vi "Inverter-data-vi.vi"() -> ()   [LabVIEW 2016]
uses:
  <vilib>/Modbus/subvis/Modbus API/Modbus API.lvclass/Modbus API.ctl
  <vilib>/Modbus/subvis/Transmission Data Unit (ADU)/Transmission Data Unit/Transmission Data Unit.lvclass/Transmission Data Unit.ctl
  <vilib>/Modbus/master/Data Access/Unit ID/Set Unit ID Property.vi
  <vilib>/Modbus/subvis/Transmission Data Unit (ADU)/Transmission Data Unit/Data Access/Unit ID/Write Unit ID.vi
  <vilib>/Modbus/subvis/Modbus API/Read Transmission Data Unit.vi
  <vilib>/Modbus/subvis/Modbus API/Write Transmission Data Unit.vi
  <vilib>/Modbus/master/Modbus Master.lvclass
  C:/Program Files (x86)/National Instruments/LabVIEW 2016/vi.lib/Modbus/subvis/Modbus API/Modbus API.lvclass
  <vilib>/Modbus/master/Create Master Instance (TCP).vi
  <vilib>/Modbus/subvis/Transmission Data Unit (ADU)/Transmission Data Unit/Transmission Data Unit.lvclass
panel:
  in  "INVERTER IP: 192.168.0.151":string
  in  "error in (no error)":errorcluster
  out "error out":errorcluster
  in  "Unit ID":u8
  in  "number of holding registers":u32
  out "BATT-TEMP":dbl
  out "DC-VOLT":dbl
  out "AC-LOAD VOLTAGE":dbl
  out "AC-LOAD-CURRENT":dbl
  out "AC-LOAD-POWER":dbl
  out "INVERTER DATA":cluster{dbl[], dbl[]}[](graph)
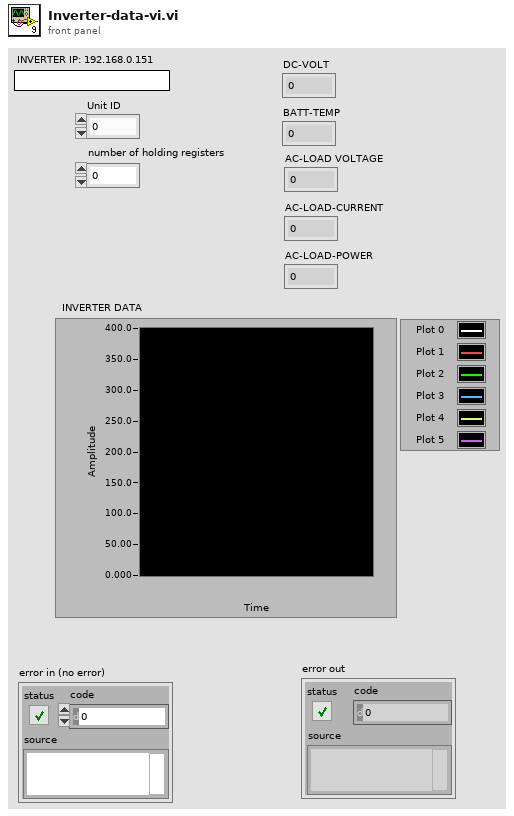
[diagram p1: front panel]
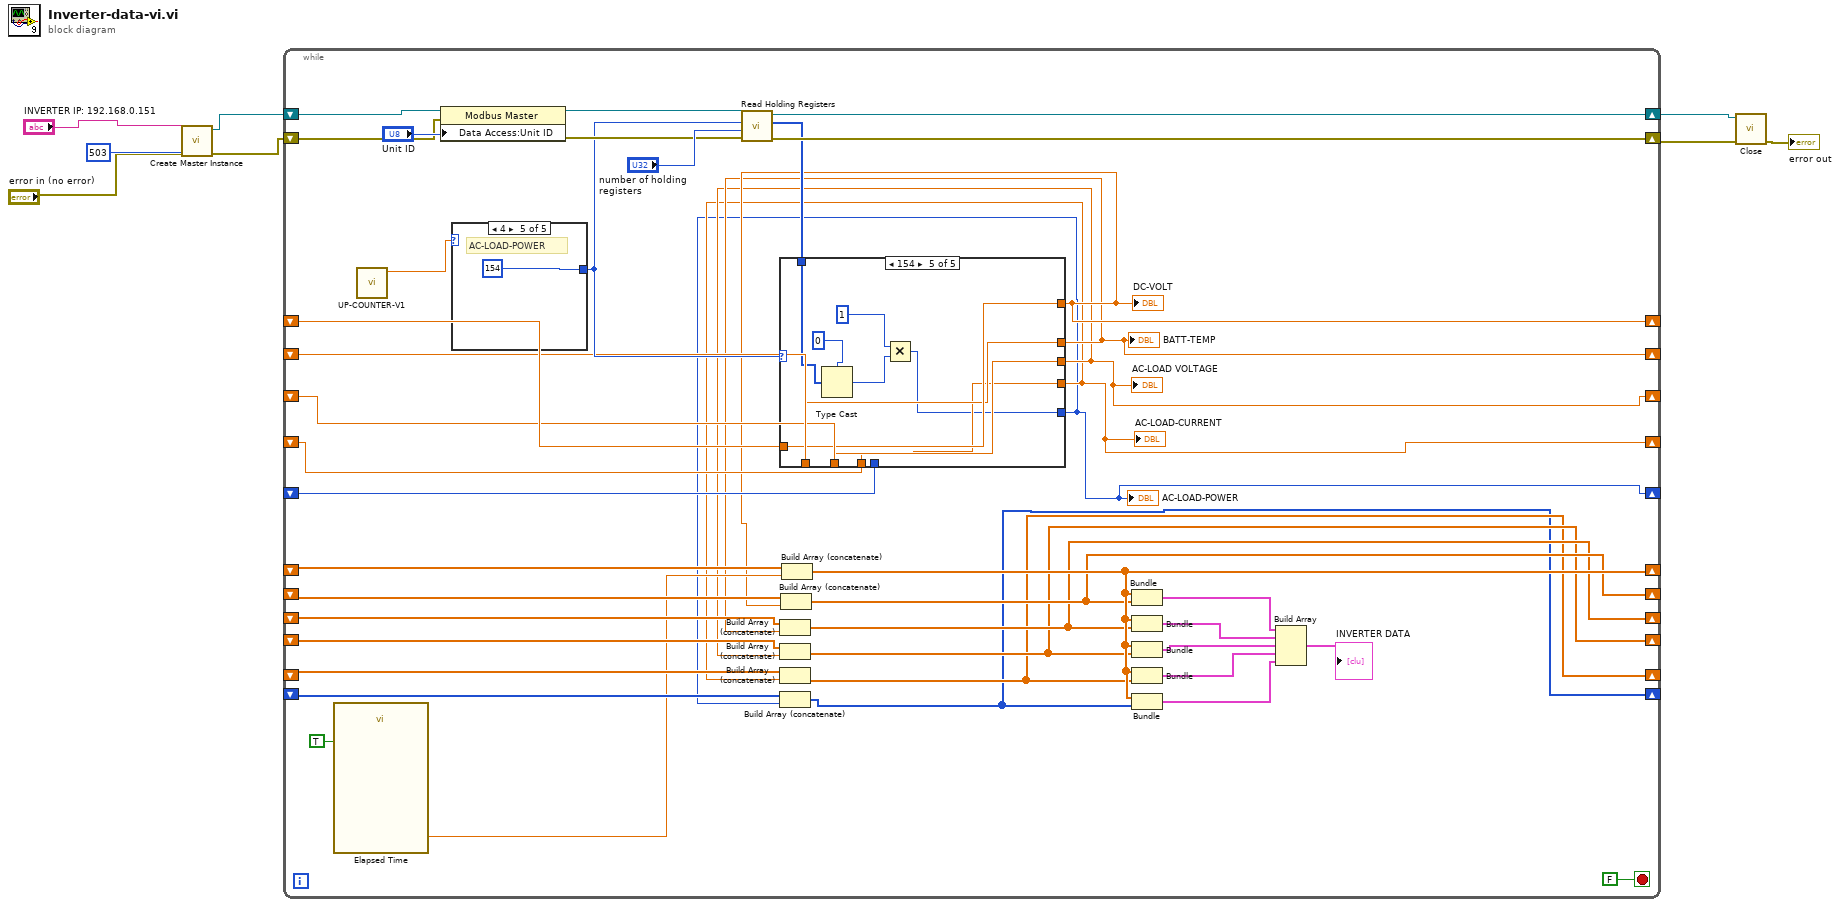
[diagram p0: block diagram]
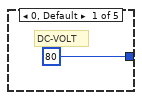
[diagram p2: hidden frame]
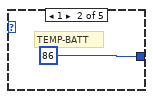
[diagram p3: hidden frame]
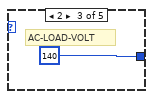
[diagram p4: hidden frame]
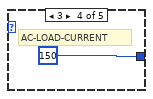
[diagram p5: hidden frame]
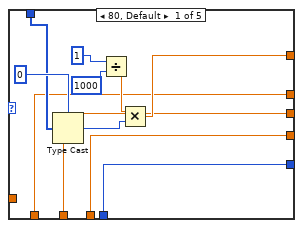
[diagram p6: hidden frame]
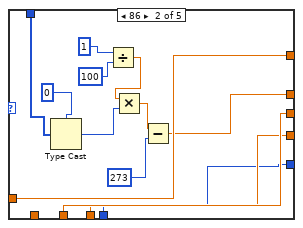
[diagram p7: hidden frame]
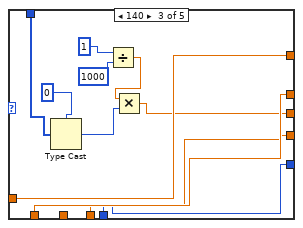
[diagram p8: hidden frame]
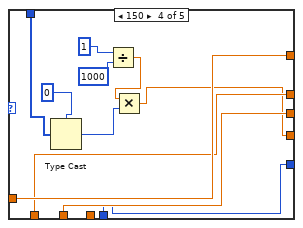
[diagram p9: hidden frame]
diagram:
  n1 = call-poly <vilib>:"Create Master Instance.vi"("error in (no error)"="error in (no error)", "port (502)"=u16 503, "address"="INVERTER IP: 192.168.0.151") -> ("error out"=w6:errorcluster, "TCP master instance"=w7:refnum<class "Modbus Master.lvclass">)  [unwired: 7 in]
  n2 = while {
    shift-right: [w48] -> w5
    shift-left: w7 -> [w50]
    shift-right: [w46] -> w4
    shift-left: w6 -> [w47]
    shift-right: [w13] -> _
    shift-left: _ -> [w38]
    shift-right: [w12] -> _
    shift-left: _ -> [w37]
    shift-right: [w11] -> _
    shift-left: _ -> [w36]
    shift-right: [w10] -> _
    shift-left: _ -> [w35]
    shift-right: [w9] -> _
    shift-left: _ -> [w34]
    shift-right: [w19] -> _
    shift-left: _ -> [w27]
    shift-right: [w18] -> _
    shift-left: _ -> [w26]
    shift-right: [w17] -> _
    shift-left: _ -> [w25]
    shift-right: [w16] -> _
    shift-left: _ -> [w24]
    shift-right: [w15] -> _
    shift-left: _ -> [w23]
    shift-right: [w14] -> _
    shift-left: _ -> [w22]
    stop <- FALSE stop-if-true
    n3 = call "Elapsed Time"("Auto Reset"=TRUE) -> ("Present (s)"=w20:dbl)  [unwired: 11 in, 7 out]
    n4 = call "UP-COUNTER-V1.vi"() -> ("COUNT"=w40:dbl)  [unwired: 11 in]
    n5 = property class="Modbus Master"(reference=w50, error in=w47, "Data Access:Unit ID"="Unit ID") -> (reference out=w41:refnum<class "Modbus Master.lvclass">, error out=w42:errorcluster)
    n6 = case shown="4" w40 {
      tunnel: [u32 80 u32 86 u32 140 u32 150 u32 154] -> w39
      frame 0, Default {
        # "DC-VOLT"
      }
      frame 1 {
        # "TEMP-BATT"
      }
      frame 2 {
        # "AC-LOAD-VOLT"
      }
      frame 3 {
        # "AC-LOAD-CURRENT"
      }
      frame 4 {
        # "AC-LOAD-POWER"
      }
    }
    n7 = call-dynamic "Read Holding Registers.vi"("error in (no error)"=w42, "number of holding registers"="number of holding registers", "starting address"=w39, "Modbus master in"=w41) -> ("error out"=w46:errorcluster, "register values"=w43:u16[], "Modbus master out"=w48:refnum<class "Modbus Master.lvclass">)  [unwired: 5 in]
    n8 = case shown="154" w39 {
      tunnel: w43 -> [w61 w70 w84 w95 w107]
      tunnel: [w60 w74 w87 w98 w110] -> w13
      tunnel: w38 -> [_ w74 w87 w98 w110]
      tunnel: [w59 w73 w83 w94 w106] -> w12
      tunnel: w37 -> [w59 _ w83 w94 w106]
      tunnel: [w58 w69 w82 w93 w105] -> w11
      tunnel: w36 -> [w58 w69 _ w93 w105]
      tunnel: [w57 w68 w81 w92 w104] -> w10
      tunnel: w35 -> [w57 w68 w81 _ w104]
      tunnel: [w56 w67 w80 w91 w103] -> w9
      tunnel: w34 -> [w56 w67 w80 w91 _]
      frame 80, Default {
        n9 = Type Cast(type=u32 0, x=w61) -> (*(type *) &x=w65:u32)
        n10 = Divide(x=u32 1, y=u32 1000) -> (x/y=w62:dbl)
        n11 = Multiply(x=w62, y=w65) -> (x*y=w60:dbl)
      }
      frame 86 {
        n12 = Type Cast(type=u16 0, x=w70) -> (*(type *) &x=w72:u16)
        n13 = Divide(x=u32 1, y=u32 100) -> (x/y=w76:dbl)
        n14 = Multiply(x=w76, y=w72) -> (x*y=w75:dbl)
        n15 = Subtract(x=w75, y=273) -> (x-y=w73:dbl)
      }
      frame 140 {
        n16 = Type Cast(type=u32 0, x=w84) -> (*(type *) &x=w86:u32)
        n17 = Divide(x=u32 1, y=u32 1000) -> (x/y=w88:dbl)
        n18 = Multiply(x=w88, y=w86) -> (x*y=w82:dbl)
      }
      frame 150 {
        n19 = Type Cast(type=0, x=w95) -> (*(type *) &x=w97:i32)
        n20 = Divide(x=u32 1, y=u32 1000) -> (x/y=w99:dbl)
        n21 = Multiply(x=w99, y=w97) -> (x*y=w92:dbl)
      }
      frame 154 {
        n22 = Type Cast(type=0, x=w107) -> (*(type *) &x=w109:i32)
        n23 = Multiply(x=1, y=w109) -> (x*y=w103:i32)
      }
    }
    "BATT-TEMP" <- w12
    "DC-VOLT" <- w13
    "AC-LOAD VOLTAGE" <- w11
    "AC-LOAD-CURRENT" <- w10
    "AC-LOAD-POWER" <- w9
    n24 = Build Array (concatenate)(w25, w12) -> (w17:dbl[])
    n25 = Build Array (concatenate)(w24, w11) -> (w16:dbl[])
    n26 = Build Array (concatenate)(w23, w10) -> (w15:dbl[])
    n27 = Build Array (concatenate)(w22, w9) -> (w14:i32[])
    n28 = Build Array (concatenate)(w26, w13) -> (w18:dbl[])
    n29 = Build Array (concatenate)(w27, w20) -> (w19:dbl[])
    n30 = Bundle(w19, w18) -> (w32:cluster{dbl[], dbl[]})  [unwired: 1 in]
    n31 = Bundle(w19, w17) -> (w31:cluster{dbl[], dbl[]})  [unwired: 1 in]
    n32 = Bundle(w19, w16) -> (w30:cluster{dbl[], dbl[]})  [unwired: 1 in]
    n33 = Bundle(w19, w15) -> (w29:cluster{dbl[], dbl[]})  [unwired: 1 in]
    n34 = Bundle(w19, w14) -> (w28:cluster{dbl[], i32[]})  [unwired: 1 in]
    n35 = Build Array(w32, w31, w30, w29, w28) -> (→"INVERTER DATA":cluster{dbl[], dbl[]}[])
  }
  n36 = call-dynamic "Close.vi"("error in (no error)"=w4, "Modbus master in"=w5) -> ("error out"=→"error out":errorcluster)  [unwired: 9 in]
